vi "Convert State Arrays to UI State-Value Pairs.vi"(10 "State Values":i32[](array[numeric]), 11 "State Names":string[](array[string])) -> (3 "Array":T1[](array[typedef]))   [LabVIEW 2017, in "Routing and Faulting System Explorer.lvlib"]
uses:
  Routing and Faulting System Explorer.lvlib
  State-Value Row.ctl
  State Control.ctl
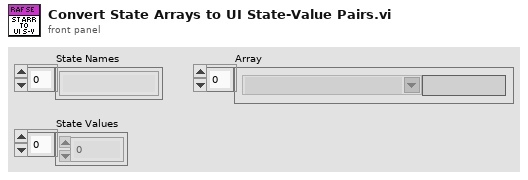
[diagram p1: front panel]
types:
  T1 = typedef "Routing and Faulting System Explorer.lvlib/State-Value Row.ctl" = cluster{"State":T2, "State Value":string}
  T2 = typedef "Routing and Faulting System Explorer.lvlib/State Control.ctl" = string
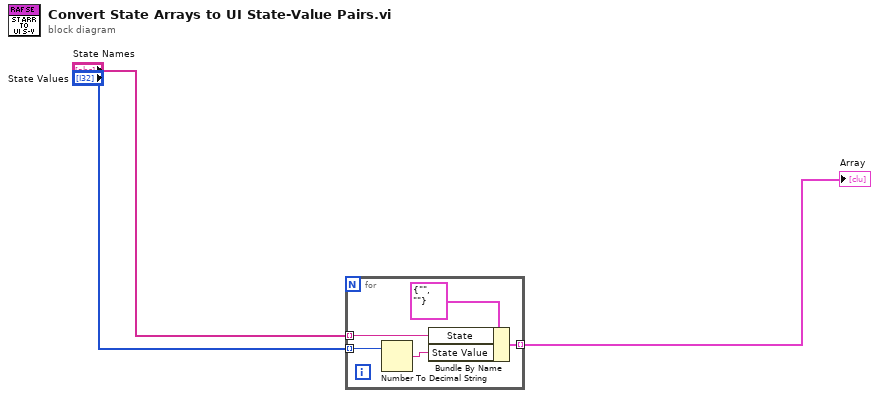
[diagram p0: block diagram]
diagram:
  n1 = for {
    tunnel: "State Names" -> [w7] mode=indexing
    tunnel: "State Values" -> [w6] mode=indexing
    tunnel: [w4] -> w3 mode=indexing
    n2 = Number To Decimal String(number=w6) -> (decimal integer string=w5:string)  [unwired: 1 in]
    n3 = Bundle By Name(cluster=T1 {"State"="", "State Value"=""} ("Alias"), "State"=w7, "State Value"=w5) -> (w4:T1)
  }
  "Array" <- w3
